vi "usrp get tx sensor.vi"(7 "sensor_value_out":u64, 8 "error in (no error)":errorcluster, 9 "chan":u64, 10 "name":string, 11 "h":u64) -> (0 "error out":errorcluster, 3 "function return":u32(ring), 5 "sensor_value_out out":u64)   [LabVIEW 2023, in "uhd.lvlib"]
doc: "UHD_API uhd_error uhd_usrp_get_tx_sensor(uhd_usrp_handle h,\n const char* name,\n size_t chan,\n uhd_sensor_value_handle* sensor_value_out);"
uses:
  <userlib>/uhd/uhd.lvlib
  <userlib>/uhd/uhd.dll
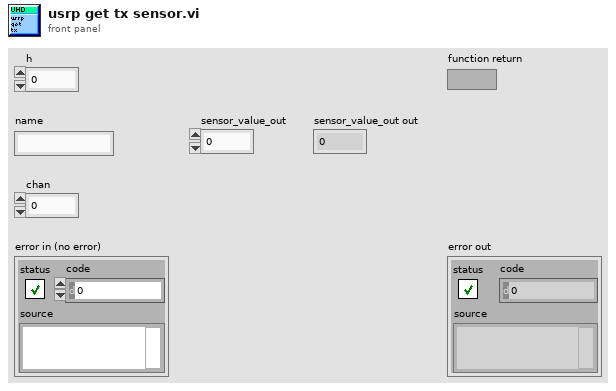
[diagram p1: front panel]
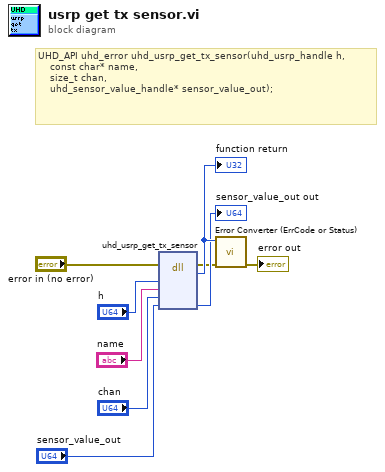
[diagram p0: block diagram]
diagram:
  # "UHD_API uhd_error uhd_usrp_get_tx_sensor(uhd_usrp_handle h,\n    const char* name,\n    size_t chan,\n    uhd_sensor_value_handle* sensor_value_out);"
  n1 = dll-call lib="C:/Program Files/National Instruments/LabVIEW 2023/user.lib/uhd/uhd.*" fn="uhd_usrp_get_tx_sensor"(error in="error in (no error)", "h"="h", "name"="name", "chan"="chan", "sensor_value_out"="sensor_value_out") -> (error out=w2:errorcluster, w9:u32, "sensor_value_out"=→"sensor_value_out out":u64)  [unwired: 5 in, 1 out]
  "function return" <- w9
  n2 = call <userlib>:"Error Converter (ErrCode or Status).vi"("error in (no error)"=w2, "error code"=w9) -> ("error out"=→"error out":errorcluster)  [unwired: 9 in]
